vi "Vision Processing Vision.vi"(4 "error in (no error)":errorcluster, 7 "Image Size":T3=enum."320x240") -> ()   [LabVIEW 2016]
doc: "This VI runs in parallel to other tasks. It gets images from the camera, processes them for color or shape and use that information to affect robot behavior."
uses:
  <vilib>/Rock Robotics/WPI/Camera/WPI_CameraImageSize.ctl
  <vilib>/Rock Robotics/WPI/Camera/WPI_CameraWhite Balance Values.ctl
  <vilib>/Rock Robotics/WPI/Camera/WPI_CameraExposure Values.ctl
  <vilib>/Rock Robotics/WPI/Camera/WPI_CameraFrameRate.ctl
  Robot Global Data.vi
panel:
  out "Image":T1(plugin-control)
  out "Number of Matches (Color Location 1)":i32
  out "Matches (calibrated) (Color Location 1)":T2(array[cluster]) {"Bounding Box"."y" format="%.2f"; "Bounding Box"."x" format="%.2f"; "Position"."y" format="%.2f"; "Position"."x" format="%.2f"; "Score" format="%.2f"; "Scale" format="%.2f"; "Angle" format="%.2f"}
  out "Matches (Color Location 1)":T2(array[cluster]) {"Bounding Box"."y" format="%.2f"; "Bounding Box"."x" format="%.2f"; "Position"."y" format="%.2f"; "Position"."x" format="%.2f"; "Score" format="%.2f"; "Scale" format="%.2f"; "Angle" format="%.2f"}
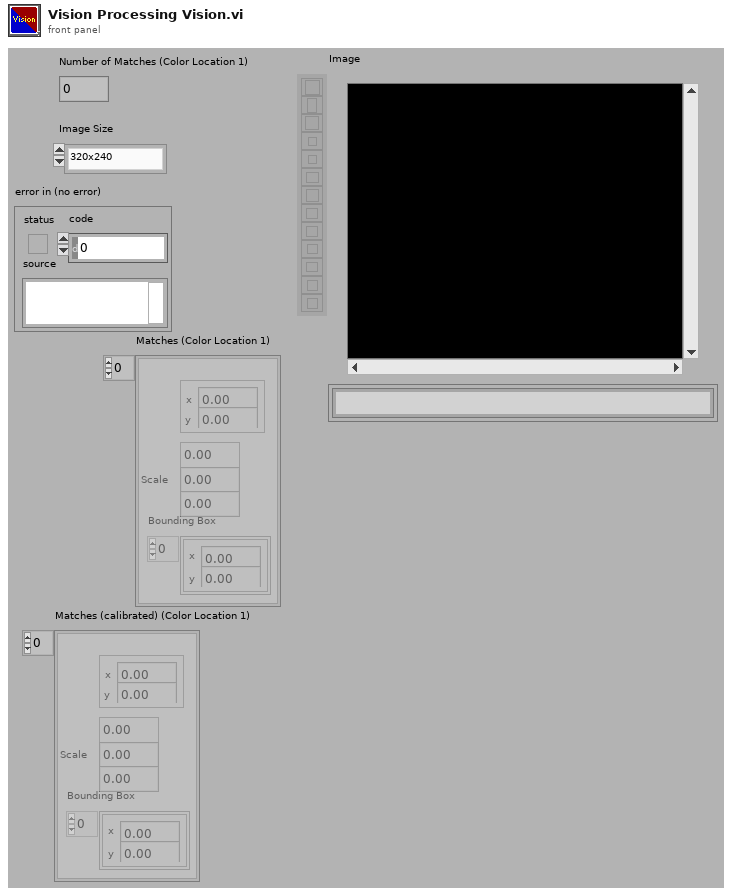
[diagram p1: front panel]
types:
  T1 = typedef "IMAQ Image.ctl" = refnum<image>
  T2 = cluster{"Position":cluster{"x":sgl, "y":sgl}, "Angle":sgl, "Scale":sgl, "Score":sgl, "Bounding Box":cluster{"x":sgl, "y":sgl}[]}[]
  T3 = typedef "WPI_CameraImageSize.ctl" = enum16{"640x480", "320x240", "160x120", "Custom"}
  T4 = typedef "WPI_CameraFrameRate.ctl" = u32
  T5 = typedef "WPI_CameraExposure Values.ctl" = enum16{"Auto", "Flicker-free 50 Hz", "Flicker-free 60 Hz", "Hold current", "Custom"}
  T6 = typedef "WPI_CameraWhite Balance Values.ctl" = enum16{"Auto", "Fixed indoor", "Fixed outdoor 1", "Fixed outdoor 2", "Fixed fluorescent 1", "Fixed fluorescent 2", "Hold current", "Custom"}
  T7 = typedef "Image Type" = u32
  T8 = typedef "WPI_CameraDevRef.ctl" = cluster{"Camera Address":string, "CameraStatus":errorcluster}
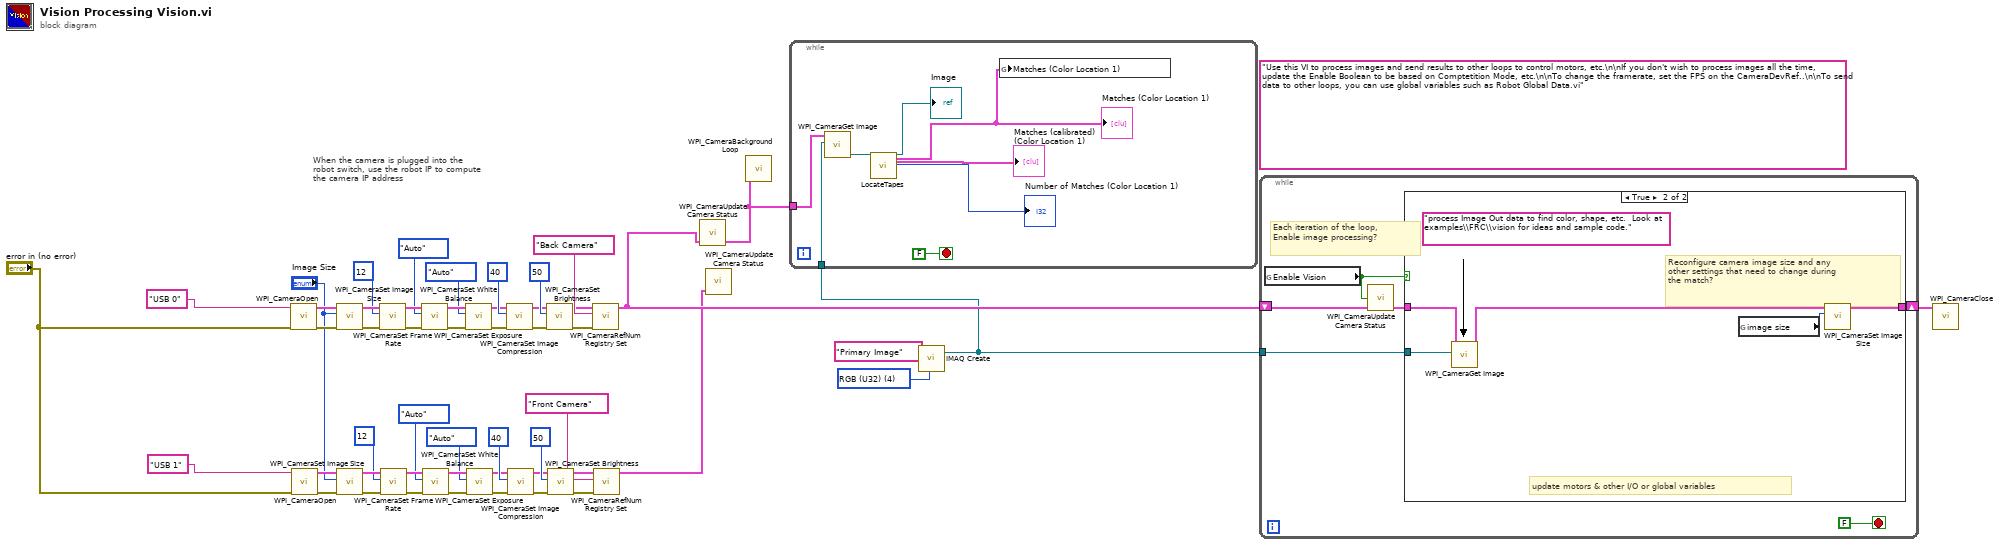
[diagram p0: block diagram]
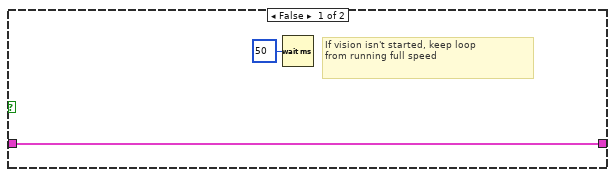
[diagram p2: hidden frame]
diagram:
  (unwired) "Use this VI to process images and send results to other loops to control motors, etc.\n\nIf you don't wish to process images all the time, update the Enable Boolean to be based on Comptetition Mode, etc.\n\nTo change the framerate, set the FPS on the CameraDevRef..\n\nTo send data to other loops, you can use global variables such as Robot Global Data.vi"
  w51 = T7 4 items=["Grayscale (U8)", "Grayscale (I16)", "Grayscale (SGL)", "Complex (CSG)", "RGB (U32)", "HSL (U32)", "RGB (U64)"] ("Image Type")
  # "When the camera is plugged into the\nrobot switch, use the robot IP to compute\nthe camera IP address"
  n1 = call <vilib>:"WPI_CameraOpen.vi"("error in (no error)"="error in (no error)", "Camera Address"="USB 0" ("format string")) -> ("error out"=w40:errorcluster, "CameraDevRef"=w41:T8)  [unwired: 8 out]
  n2 = call <vilib>:"WPI_CameraOpen.vi"("error in (no error)"="error in (no error)", "Camera Address"="USB 1" ("format string")) -> ("error out"=w19:errorcluster, "CameraDevRef"=w20:T8)  [unwired: 8 out]
  n3 = call <vilib>:"WPI_CameraSet Image Size.vi"("error in (no error)"=w40, "Image Size"="Image Size", "CameraDevRef"=w41) -> ("error out"=w39:errorcluster, "CameraDevRef Out"=w42:T8)  [unwired: 1 in, 6 out]
  n4 = call <vilib>:"WPI_CameraSet Image Size.vi"("error in (no error)"=w19, "Image Size"="Image Size", "CameraDevRef"=w20) -> ("error out"=w18:errorcluster, "CameraDevRef Out"=w21:T8)  [unwired: 1 in, 6 out]
  n5 = call <vilib>:"WPI_CameraSet Frame Rate.vi"("error in (no error)"=w39, "Frame Rate (fps)"=T4 12, "CameraDevRef"=w42) -> ("error out"=w38:errorcluster, "CameraDevRef Out"=w44:T8)  [unwired: 7 out]
  n6 = call <vilib>:"WPI_CameraSet Frame Rate.vi"("error in (no error)"=w18, "Frame Rate (fps)"=T4 12, "CameraDevRef"=w21) -> ("error out"=w17:errorcluster, "CameraDevRef Out"=w23:T8)  [unwired: 7 out]
  n7 = call <vilib>:"WPI_CameraSet White Balance.vi"("error in (no error)"=w38, "White Balance"=WPI_CameraWhite_Balance_Values."Auto", "CameraDevRef"=w44) -> ("error out"=w37:errorcluster, "CameraDevRef Out"=w43:T8)  [unwired: 1 in, 6 out]
  n8 = call <vilib>:"WPI_CameraSet White Balance.vi"("error in (no error)"=w17, "White Balance"=WPI_CameraWhite_Balance_Values."Auto", "CameraDevRef"=w23) -> ("error out"=w16:errorcluster, "CameraDevRef Out"=w22:T8)  [unwired: 1 in, 6 out]
  n9 = call <vilib>:"WPI_CameraSet Exposure.vi"("error in (no error)"=w37, "Exposure"=WPI_CameraExposure_Values."Auto", "CameraDevRef"=w43) -> ("error out"=w36:errorcluster, "CameraDevRef Out"=w46:T8)  [unwired: 1 in, 6 out]
  n10 = call <vilib>:"WPI_CameraSet Exposure.vi"("error in (no error)"=w16, "Exposure"=WPI_CameraExposure_Values."Auto", "CameraDevRef"=w22) -> ("error out"=w15:errorcluster, "CameraDevRef Out"=w25:T8)  [unwired: 1 in, 6 out]
  n11 = call <vilib>:"WPI_CameraSet Image Compression.vi"("error in (no error)"=w36, "Compression"=40, "CameraDevRef"=w46) -> ("error out"=w35:errorcluster, "CameraDevRef Out"=w45:T8)  [unwired: 7 out]
  n12 = call <vilib>:"WPI_CameraSet Image Compression.vi"("error in (no error)"=w15, "Compression"=40, "CameraDevRef"=w25) -> ("error out"=w14:errorcluster, "CameraDevRef Out"=w24:T8)  [unwired: 7 out]
  n13 = call <vilib>:"WPI_CameraSet Brightness.vi"("error in (no error)"=w35, "Brightness"=50, "CameraDevRef"=w45) -> ("error out"=w33:errorcluster, "CameraDevRef Out"=w34:T8)  [unwired: 7 out]
  n14 = call <vilib>:"WPI_CameraSet Brightness.vi"("error in (no error)"=w14, "Brightness"=50, "CameraDevRef"=w24) -> ("error out"=w12:errorcluster, "CameraDevRef Out"=w13:T8)  [unwired: 7 out]
  n15 = call <vilib>:"WPI_CameraRefNum Registry Set.vi"("error in (no error)"=w33, "refnum name"="Back Camera", "CameraDevRef"=w34) -> ("CameraDevRef"=w4:T8)  [unwired: 1 in, 7 out]
  n16 = call <vilib>:"WPI_CameraRefNum Registry Set.vi"("error in (no error)"=w12, "refnum name"="Front Camera", "CameraDevRef"=w13) -> ("CameraDevRef"=w3:T8)  [unwired: 1 in, 7 out]
  n17 = call <vilib>:"WPI_CameraUpdate Camera Status.vi"("CameraDevRef In"=w4) -> ("CameraDevRef Out"=w2:T8)  [unwired: 4 in]
  n18 = call <vilib>:"WPI_CameraUpdate Camera Status.vi"("CameraDevRef In"=w3) -> ()  [unwired: 4 in, 1 out]
  n19 = call <vilib>:"WPI_CameraBackground Loop.vi"("CameraDevRef"=w2) -> ()  [unwired: 11 in]
  n20 = call "IMAQ Create"("Image Name"="Primary Image", "Image Type"=w51) -> ("New Image"=w1:T1)  [unwired: 2 in, 2 out]
  n21 = while {
    tunnel: w2 -> [w58]
    tunnel: w1 -> [w54]
    stop <- FALSE stop-if-true
    n22 = call <vilib>:"WPI_CameraGet Image.vi"("Image"=w54, "CameraDevRef"=w58) -> ("Image Out"=w57:T1)  [unwired: 7 in, 2 out]
    n23 = call "LocateTapes.vi"("Image In"=w57) -> ("Image Out"=→"Image":T1, "Matches (Color Location 1)"=w52:T2, "Matches (calibrated) (Color Location 1)"=→"Matches (calibrated) (Color Location 1)":T2, "Number of Matches (Color Location 1)"=→"Number of Matches (Color Location 1)":i32)  [unwired: 22 in, 1 out]
    "Matches (Color Location 1)" <- w52
    n24 = global write "Robot Global Data.vi" "Matches (Color Location 1)"(w52) -> ()
  }
  n25 = while {
    shift-right: [w64] -> w29
    shift-left: w4 -> [w62]
    tunnel: w1 -> [w63]
    stop <- FALSE stop-if-true
    # "Each iteration of the loop,\nEnable image processing?"
    n26 = global read "Robot Global Data.vi" "Enable Vision"() -> (w60:bool)
    n27 = call <vilib>:"WPI_CameraUpdate Camera Status.vi"("CameraDevRef In"=w62, "Enable Vision"=w60) -> ("CameraDevRef Out"=w61:T8)  [unwired: 3 in]
    n28 = case shown="True" w60 {
      tunnel: w63 -> [_ w71]
      tunnel: [w67 w72] -> w64
      tunnel: w61 -> [w67 w69]
      frame False {
        # "If vision isn't started, keep loop\nfrom running full speed"
        n29 = Wait (ms)(milliseconds to wait=u32 50) -> ()  [unwired: 1 out]
      }
      frame True {
        (unwired) "process Image Out data to find color, shape, etc.  Look at examples\\FRC\\vision for ideas and sample code."
        # "update motors & other I/O or global variables"
        # "Reconfigure camera image size and any\nother settings that need to change during\nthe match?"
        n30 = call <vilib>:"WPI_CameraGet Image.vi"("Image"=w71, "CameraDevRef"=w69) -> ("CameraDevRef Out"=w68:T8)  [unwired: 1 in, 8 out]
        n31 = global read "Robot Global Data.vi" "image size"() -> (w70:T3)
        n32 = call <vilib>:"WPI_CameraSet Image Size.vi"("Image Size"=w70, "CameraDevRef"=w68) -> ("CameraDevRef Out"=w72:T8)  [unwired: 2 in, 7 out]
      }
    }
  }
  n33 = call <vilib>:"WPI_CameraClose.vi"("CameraDevRef"=w29) -> ()  [unwired: 1 in, 10 out]
